vi "HexString_To_U16.vi"(10 "Position":i32, 11 "String":string) -> (3 "U16":u32)   [LabVIEW 2015]
doc: "Selects a substring and convert it to a hex U16.\n\nString position starts with 0"
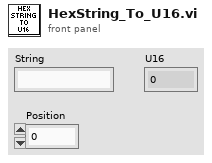
[diagram p1: front panel]
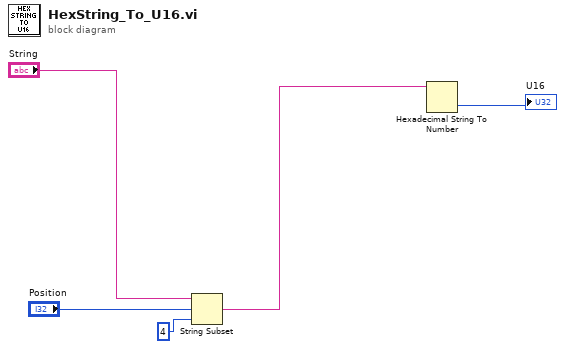
[diagram p0: block diagram]
diagram:
  n1 = String Subset(string="String", offset (0)="Position", length (rest)=4 ("length (rest)")) -> (substring=w1:string)
  n2 = Hexadecimal String To Number(string=w1) -> (number=→"U16":u32)  [unwired: 2 in, 1 out]
